vi "Send SCPI Strings.vi"(1 "Check For SCPI Errors? (T)":bool=TRUE, 5 "SCPI Strings (no term char)":string[](array[string]), 9 "Num Bytes To Read (256)":u32=256, 14 "Trim End Whitespace? (T)":bool=TRUE) -> (4 "Resource Out (dupl)":refnum<visa-resource-name>, 6 "Query Responses":string[](array[string]), 8 "Num Strings Sent":i32)   [LabVIEW 2016, in "Keithley 622x.lvlib"]
uses:
  Keithley 622x.lvlib
  <vilib>/Utility/error.llb/whitespace.ctl
panel:
  out "error out 2":errorcluster
  in  "Port":string
  in  "IP":string
  out "Numeric":i32
  in  "stop":bool
  # "^"
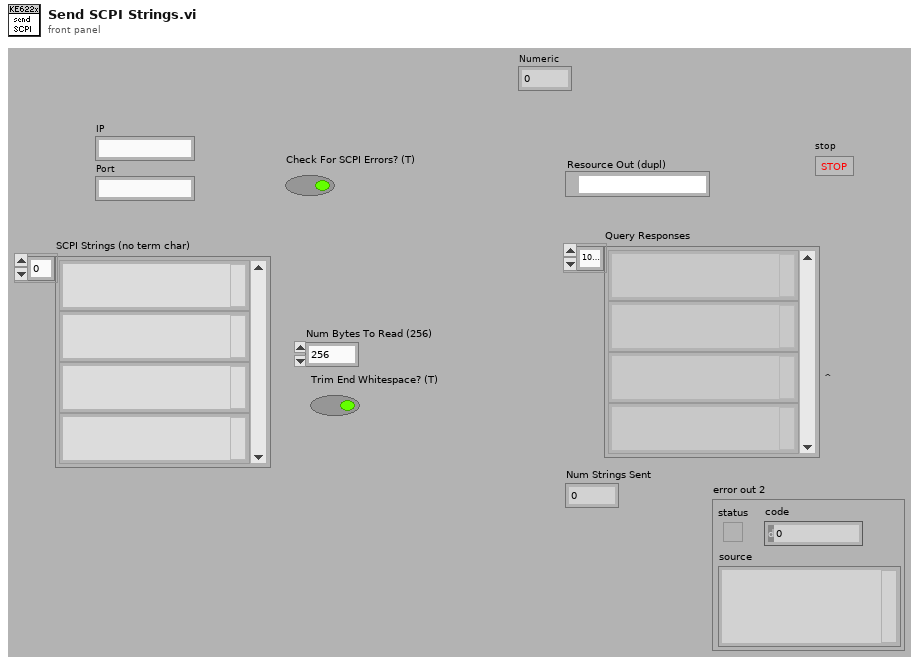
[diagram p1: front panel]
types:
  T1 = typedef "whitespace.ctl" = u16
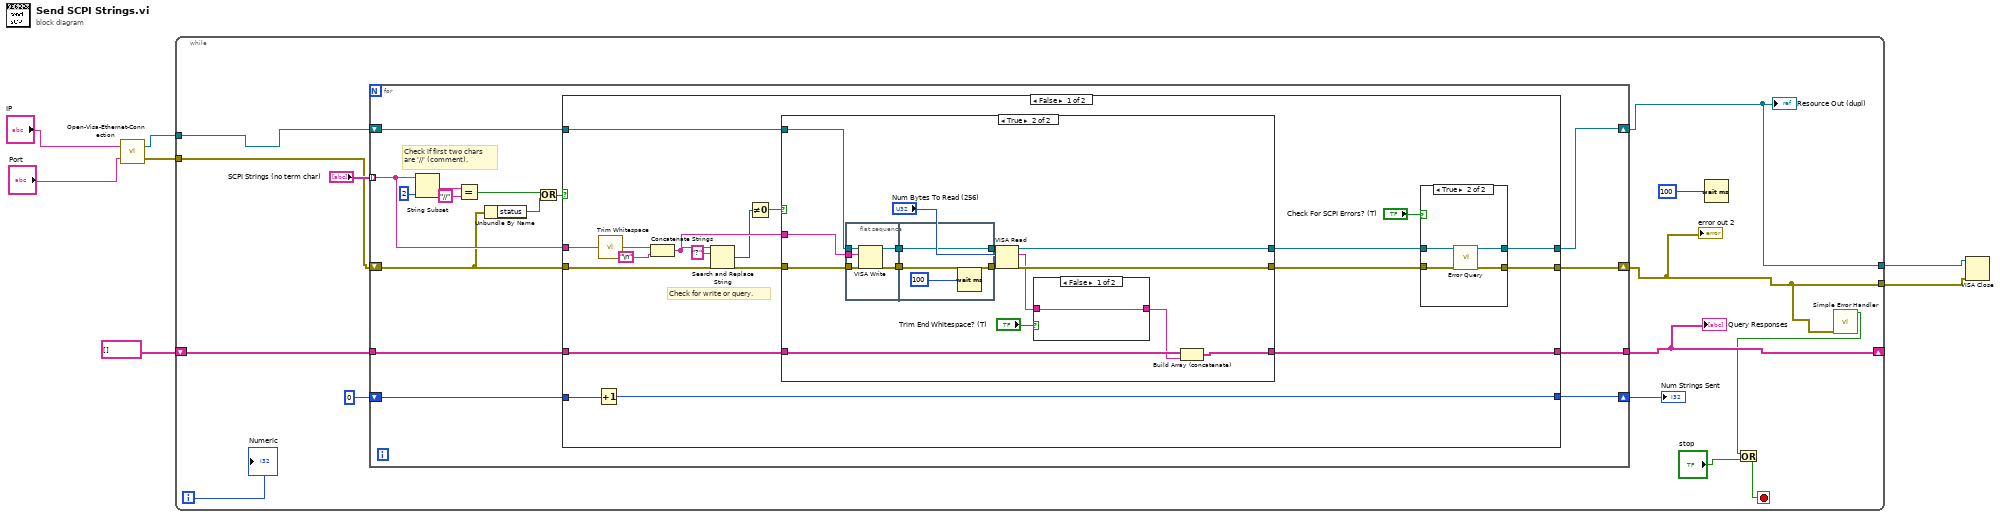
[diagram p0: block diagram]
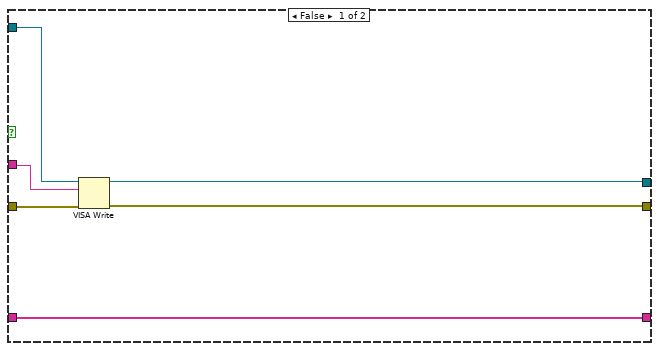
[diagram p3: hidden frame]
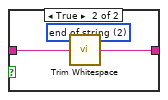
[diagram p4: hidden frame]
diagram:
  n1 = call "Open-Visa-Ethernet-Connection.vi"("Port"="Port", "IP"="IP") -> ("error out"=w3:errorcluster, "VISA resource name out"=w4:refnum<visa-resource-name>)
  n2 = while {
    shift-right: [w15] -> _
    shift-left: string[] [] -> [w16]
    tunnel: w4 -> [w13]
    tunnel: w3 -> [w14]
    tunnel: [w11] -> w2
    tunnel: [w12] -> w1
    i -> [w17]
    stop <- w8 stop-if-true
    n3 = for {
      tunnel: "SCPI Strings (no term char)" -> [w32] mode=indexing
      shift-right: [w28] -> w11
      shift-left: w14 -> [w26]
      shift-right: [w27] -> w12
      shift-left: w13 -> [w31]
      shift-right: [w22] -> w19
      shift-left: 0 -> [w23]
      tunnel: w16 -> [w30]
      tunnel: [w29] -> w15
      # "Check if first two chars\nare '//' (comment)."
      n4 = String Subset(string=w32, length (rest)=2 ("length (rest)")) -> (substring=w35:string)  [unwired: 1 in]
      n5 = Equal?(x=w35, y="//") -> (x = y?=w33:bool)
      n6 = Unbundle By Name(w26) -> ("status"=w24:bool)
      n7 = Or(x=w33, y=w24) -> (x .or. y?=w25:bool)
      n8 = case shown="False" w25 {
        tunnel: w26 -> [w55 w97]
        tunnel: w32 -> [w54 _]
        tunnel: w31 -> [w50 w96]
        tunnel: w30 -> [w48 w98]
        tunnel: [w47 w98] -> w29
        tunnel: [w43 w97] -> w28
        tunnel: [w42 w96] -> w27
        tunnel: w23 -> [w41 w95]
        tunnel: [w40 w95] -> w22
        frame False {
          # "Check for write or query."
          n9 = Increment(x=w41) -> (x+1=w40:i32)
          n10 = call <vilib>:"Trim Whitespace.vi"("string"=w54) -> ("trimmed string"=w39:string)  [unwired: 1 in]
          n11 = Concatenate Strings(w39, "\n") -> (w49:string)
          n12 = Search and Replace String(input string=w49, search string="?", error in=w55) -> (number of replacements=w38:i32, error out=w51:errorcluster)  [unwired: 5 in, 2 out]
          n13 = Not Equal To 0?(x=w38) -> (x != 0?=w52:bool)
          n14 = case shown="True" w52 {
            tunnel: w51 -> [w66 w82]
            tunnel: w50 -> [w64 w81]
            tunnel: w49 -> [w65 w80]
            tunnel: [w62 w76] -> w45
            tunnel: [w63 w75] -> w44
            tunnel: w48 -> [w67 w72]
            tunnel: [w67 w70] -> w47
            frame False {
              n15 = VISA Write(VISA resource name=w64, write buffer=w65, error in (no error)=w66) -> (VISA resource name out=w62:refnum<visa-resource-name>, error out=w63:errorcluster)  [unwired: 1 out]
            }
            frame True {
              n16 = flat-sequence {
                tunnel: w82 -> [w87]
                tunnel: w81 -> [w86]
                tunnel: w80 -> [w85]
                tunnel: [w84] -> w69
                tunnel: [w83] -> w68
                tunnel: [w89] -> w77
                tunnel: [w90] -> w78
                tunnel: w69 -> [w90]
                tunnel: w68 -> [w89]
                frame #0 {
                  n17 = VISA Write(VISA resource name=w86, write buffer=w85, error in (no error)=w87) -> (VISA resource name out=w84:refnum<visa-resource-name>, error out=w83:errorcluster)  [unwired: 1 out]
                }
                frame #1 {
                  n18 = Wait (ms)(milliseconds to wait=100) -> ()  [unwired: 1 out]
                }
              }
              n19 = VISA Read(VISA resource name=w78, byte count="Num Bytes To Read (256)", error in (no error)=w77) -> (VISA resource name out=w76:refnum<visa-resource-name>, read buffer=w73:string, error out=w75:errorcluster)  [unwired: 1 out]
              n20 = case shown="False" "Trim End Whitespace? (T)" {
                tunnel: w73 -> [w91 w93]
                tunnel: [w91 w92] -> w71
                frame False {
                }
                frame True {
                  w94 = T1 2 items=["both", "start of string", "end of string"] ("location (both)")
                  n21 = call <vilib>:"Trim Whitespace.vi"("string"=w93, "location (both)"=w94) -> ("trimmed string"=w92:string)
                }
              }
              n22 = Build Array (concatenate)(w72, w71) -> (w70:string[])
            }
          }
          n23 = case shown="True" "Check For SCPI Errors? (T)" {
            tunnel: w45 -> [w57 w61]
            tunnel: w44 -> [w56 w60]
            tunnel: [w56 w59] -> w43
            tunnel: [w57 w58] -> w42
            frame False {
            }
            frame True {
              n24 = call "Error Query.vi"("VISA Resource In"=w61, "error in (no error)"=w60) -> ("VISA Resource Out (dupl)"=w58:refnum<visa-resource-name>, "error out"=w59:errorcluster)  [unwired: 10 in, 2 out]
            }
          }
        }
        frame True {
          # "Comment (or commented out), or error, so don't do anything."
        }
      }
    }
    "Num Strings Sent" <- w19
    "Query Responses" <- w15
    "error out 2" <- w11
    "Resource Out (dupl)" <- w12
    n25 = Wait (ms)(milliseconds to wait=100) -> ()  [unwired: 1 out]
    n26 = call <vilib>:"Simple Error Handler.vi"("error in (no error)"=w11) -> ("error?"=w9:bool)  [unwired: 4 in, 4 out]
    n27 = Or(x=w9, y="stop") -> (x .or. y?=w8:bool)
    "Numeric" <- w17
  }
  n28 = VISA Close(VISA resource name=w1, error in (no error)=w2) -> ()  [unwired: 1 out]
